vi "Generator.GetQueueStatus.vi"(8 "error in (no error)":errorcluster, 11 "Generator in":refnum<class "Generator.lvclass">) -> (0 "error out":errorcluster, 2 "# elements":i32, 3 "Generator out":refnum<class "Generator.lvclass">)   [LabVIEW 2019, in "Generator.lvclass"]
uses:
  Generator.lvclass
  Generator.lvclass/Generator.ctl
panel:
  out "AO Queue Refnum":i32
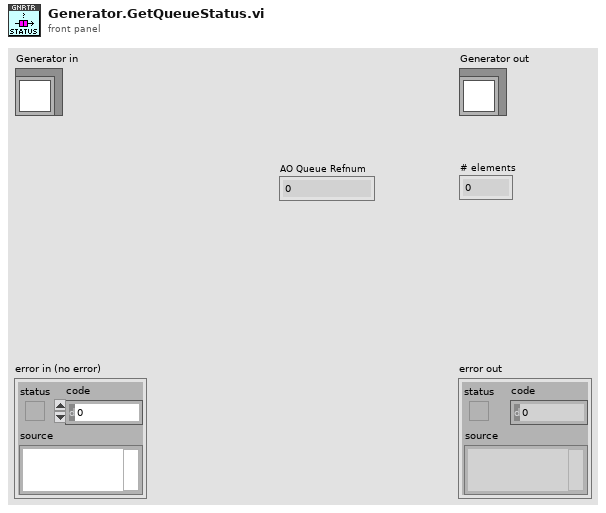
[diagram p1: front panel]
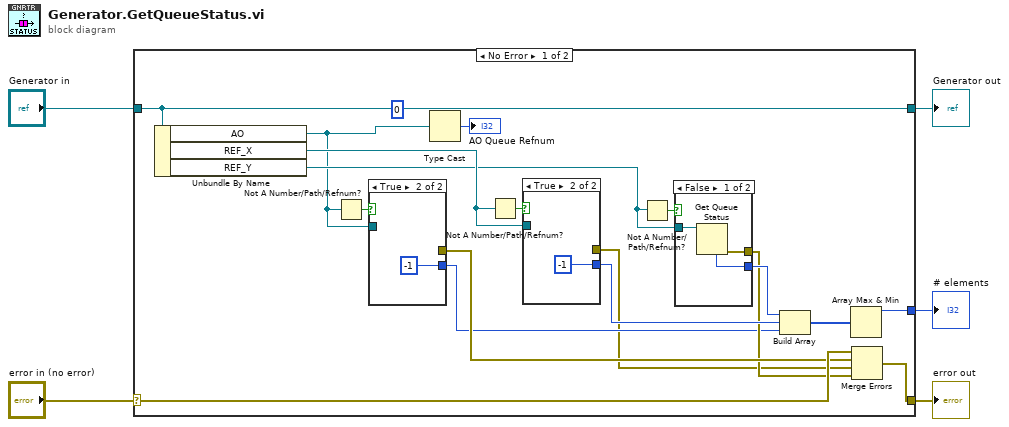
[diagram p0: block diagram]
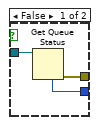
[diagram p2: hidden frame]
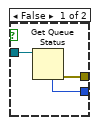
[diagram p3: hidden frame]
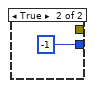
[diagram p4: hidden frame]
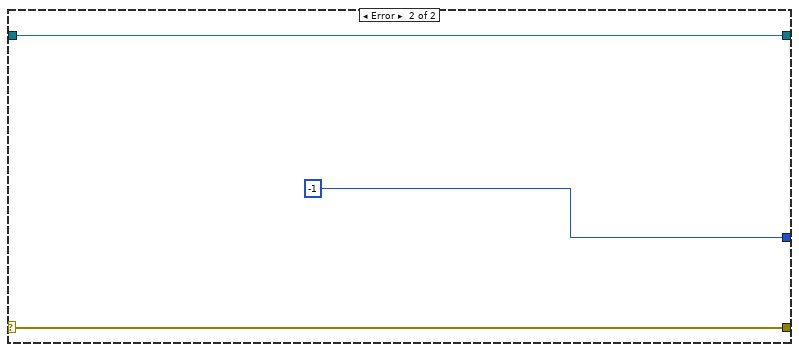
[diagram p5: hidden frame]
diagram:
  n1 = case shown="No Error" "error in (no error)" {
    selector: "error in (no error)" -> [w23 w39]
    tunnel: [w22 w39] -> w4
    tunnel: [w17 w38] -> w2
    tunnel: "Generator in" -> [w17 w38]
    tunnel: [w24 -1] -> w1
    frame No Error {
      n2 = Unbundle By Name(w17) -> ("AO"=w7:refnum<queue>, "REF_X"=w13:refnum<queue>, "REF_Y"=w12:refnum<queue>)
      n3 = Not A Number/Path/Refnum?(number/path/refnum=w7) -> (NaN/Path/Refnum?=w21:bool)
      n4 = case shown="True" w21 {
        tunnel: w7 -> [w27 _]
        tunnel: [w26 -1] -> w10
        tunnel: [w25 _] -> w20
        frame False {
          n5 = Get Queue Status(queue=w27) -> (error out=w25:errorcluster, # elements in queue=w26:i32)  [unwired: 2 in, 6 out]
        }
        frame True {
        }
      }
      n6 = Type Cast(type=0, x=w7) -> (*(type *) &x=→"AO Queue Refnum":i32)
      n7 = Not A Number/Path/Refnum?(number/path/refnum=w13) -> (NaN/Path/Refnum?=w19:bool)
      n8 = case shown="True" w19 {
        tunnel: w13 -> [w31 _]
        tunnel: [w30 -1] -> w15
        tunnel: [w29 _] -> w9
        frame False {
          n9 = Get Queue Status(queue=w31) -> (error out=w29:errorcluster, # elements in queue=w30:i32)  [unwired: 2 in, 6 out]
        }
        frame True {
        }
      }
      n10 = Not A Number/Path/Refnum?(number/path/refnum=w12) -> (NaN/Path/Refnum?=w18:bool)
      n11 = case shown="False" w18 {
        tunnel: w12 -> [w35 _]
        tunnel: [w34 -1] -> w16
        tunnel: [w33 _] -> w11
        frame False {
          n12 = Get Queue Status(queue=w35) -> (error out=w33:errorcluster, # elements in queue=w34:i32)  [unwired: 2 in, 6 out]
        }
        frame True {
        }
      }
      n13 = Build Array(w16, w15, w10) -> (w14:i32[])
      n14 = Array Max & Min(array=w14) -> (max value=w24:i32)  [unwired: 3 out]
      n15 = Merge Errors(w23, w20, w9, w11) -> (w22:errorcluster)
    }
    frame Error {
    }
  }
  "error out" <- w4
  "Generator out" <- w2
  "# elements" <- w1
